vi "Clear Rx Data Available.vi"(8 "error in (no error)":errorcluster, 9 "Rx SubAddress (1-30)":u16, 10 "RT1?":bool, 11 "1553 Component in":refnum<class "1553 Component.lvclass">) -> (0 "error out":errorcluster, 3 "1553 Component out":refnum<class "1553 Component.lvclass">)   [LabVIEW 2020, in "BCI-1553 API.lvlib" / "1553 Component.lvclass"]
doc: "Attempts to clear the flag raised for new data received by the target subaddress. If the subcomponent is not an RT, the method will return an error. On success, this method will reset the data available flag and allow for the detection of another data receive event."
uses:
  1553 Component.lvclass
  1553 Component.lvclass/1553 Component.ctl
  Remote Terminal/Remote Terminal.lvclass
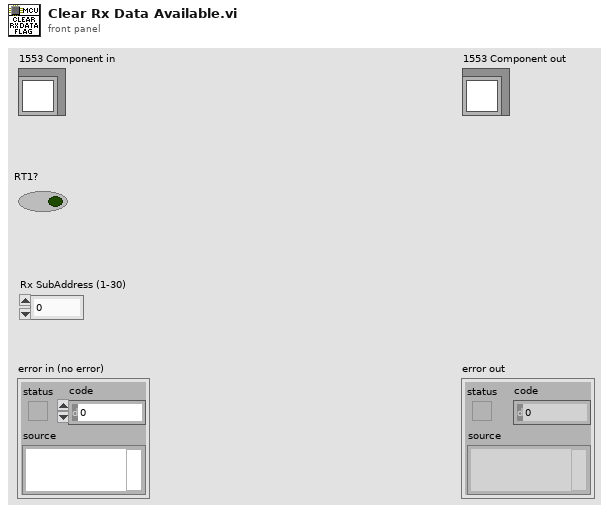
[diagram p1: front panel]
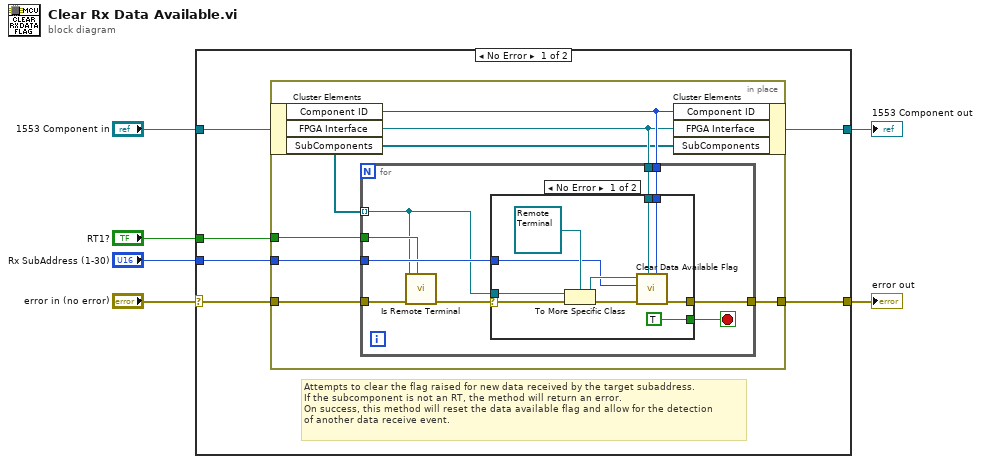
[diagram p0: block diagram]
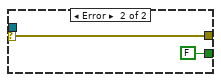
[diagram p2: hidden frame]
diagram:
  n1 = case shown="No Error" "error in (no error)" {
    selector: "error in (no error)" -> [w9 w42]
    tunnel: [w8 w42] -> w1
    tunnel: [w11 w41] -> w2
    tunnel: "1553 Component in" -> [w12 w41]
    tunnel: "Rx SubAddress (1-30)" -> [w10 _]
    tunnel: "RT1?" -> [w7 _]
    frame No Error {
      # "Attempts to clear the flag raised for new data received by the target subaddress. \nIf the subcomponent is not an RT, the method will return an error.\nOn success, this method will reset the data available flag and allow for the detection\nof another data receive event."
      n2 = in-place {
        in-place-border: w9 -> [w16]
        in-place-border: [w17] -> w8
        in-place-border: w7 -> [w14]
        in-place-border: w10 -> [w15]
        n3 = in-place-cluster #1(w12) -> ("Component ID"=w19:u8, "FPGA Interface"=w18:refnum<class "FPGA Interface.lvclass">, "SubComponents"=w13:refnum<class "1553 SubComponent.lvclass">[])
        n4 = for {
          tunnel: w19 -> [w28]
          tunnel: w18 -> [w27]
          tunnel: w15 -> [w23]
          tunnel: w14 -> [w22]
          tunnel: w13 -> [w21] mode=indexing
          tunnel: w16 -> [w25]
          tunnel: [w26] -> w17
          stop <- w20 stop-if-true
          n5 = call "Is Remote Terminal.vi"("RT1?"=w22, "error in (no error)"=w25, "1553 SubComponent"=w21) -> ("error out"=w24:errorcluster)  [unwired: 8 in]
          n6 = case shown="No Error" w24 {
            selector: w24 -> [w37 w40]
            tunnel: w28 -> [w31 _]
            tunnel: w27 -> [w32 _]
            tunnel: [w30 w40] -> w26
            tunnel: w21 -> [w38 _]
            tunnel: w23 -> [w34 _]
            tunnel: [TRUE FALSE] -> w20
            frame No Error {
              n7 = To More Specific Class(target class=refnum<class "Remote Terminal.lvclass"> refnum ("SLSC 1553 API.lvlib:Remote Terminal.lvclass"), reference=w38, error in=w37) -> (specific class reference=w36:refnum<class "Remote Terminal.lvclass">, error out=w33:errorcluster)
              n8 = call-dynamic "Clear Data Available Flag.vi"("Component ID"=w31, "FPGA Interface"=w32, "error in (no error)"=w33, "Rx SubAddress (1-30)"=w34, "Remote Terminal in"=w36) -> ("error out"=w30:errorcluster)  [unwired: 6 in]
            }
            frame Error {
            }
          }
        }
        n9 = in-place-cluster #1("Component ID"=w19, "FPGA Interface"=w18, "SubComponents"=w13) -> (w11:refnum<class "1553 Component.lvclass">)
      }
    }
    frame Error {
    }
  }
  "error out" <- w1
  "1553 Component out" <- w2
